vi "UUT Test Info Update Cycle Count.vi"(11 "Sequence Context":T1) -> (0 "error out":errorcluster)   [LabVIEW 2023, in "HardwareAbstractionLayer_LVOOP.lvlib" / "Report.lvclass"]
uses:
  Report.lvclass
  <vilib>/addons/TestStand/_TSLegacy.llb/LabVIEW Test - Sequence Context.ctl
  Database/SQL Public VI/Control/DB Options.ctl
  <vilib>/addons/TestStand/_TSUtility.llb/TestStand - Get Property Value (Number {Unsigned 32-bit Integer}).vi
  Database/Database.lvclass
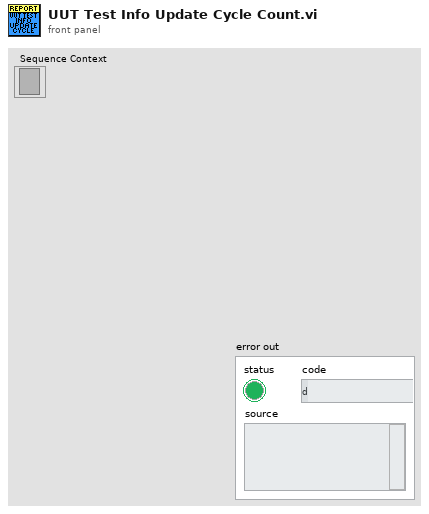
[diagram p1: front panel]
types:
  T1 = typedef "LabVIEW Test - Sequence Context.ctl" = refnum<k7>
  T2 = typedef "HardwareAbstractionLayer_LVOOP.lvlib/Database.lvclass/DB Options.ctl" = enum16{"Init", "Select Data", "Insert Data", "Update Data", "Delete Data", "Execute Query", "Create Schema", "Create Table", "List Tables", "List Columns", "Close"}
  T3 = typedef "HardwareAbstractionLayer_LVOOP.lvlib/Report.lvclass/Result FGV Data.ctl" = cluster{"Project Name":string, "Product Name":string, "Product Varient":string, "Test Name":string, "Test Phase":string, "Test Description":string, "Temp Chamber Name":string, "Schema":string, "Total No of Cycles":u32, "Current Cycle Number":u32, "Cycle Duration":u32, "Current Test Mode":string}
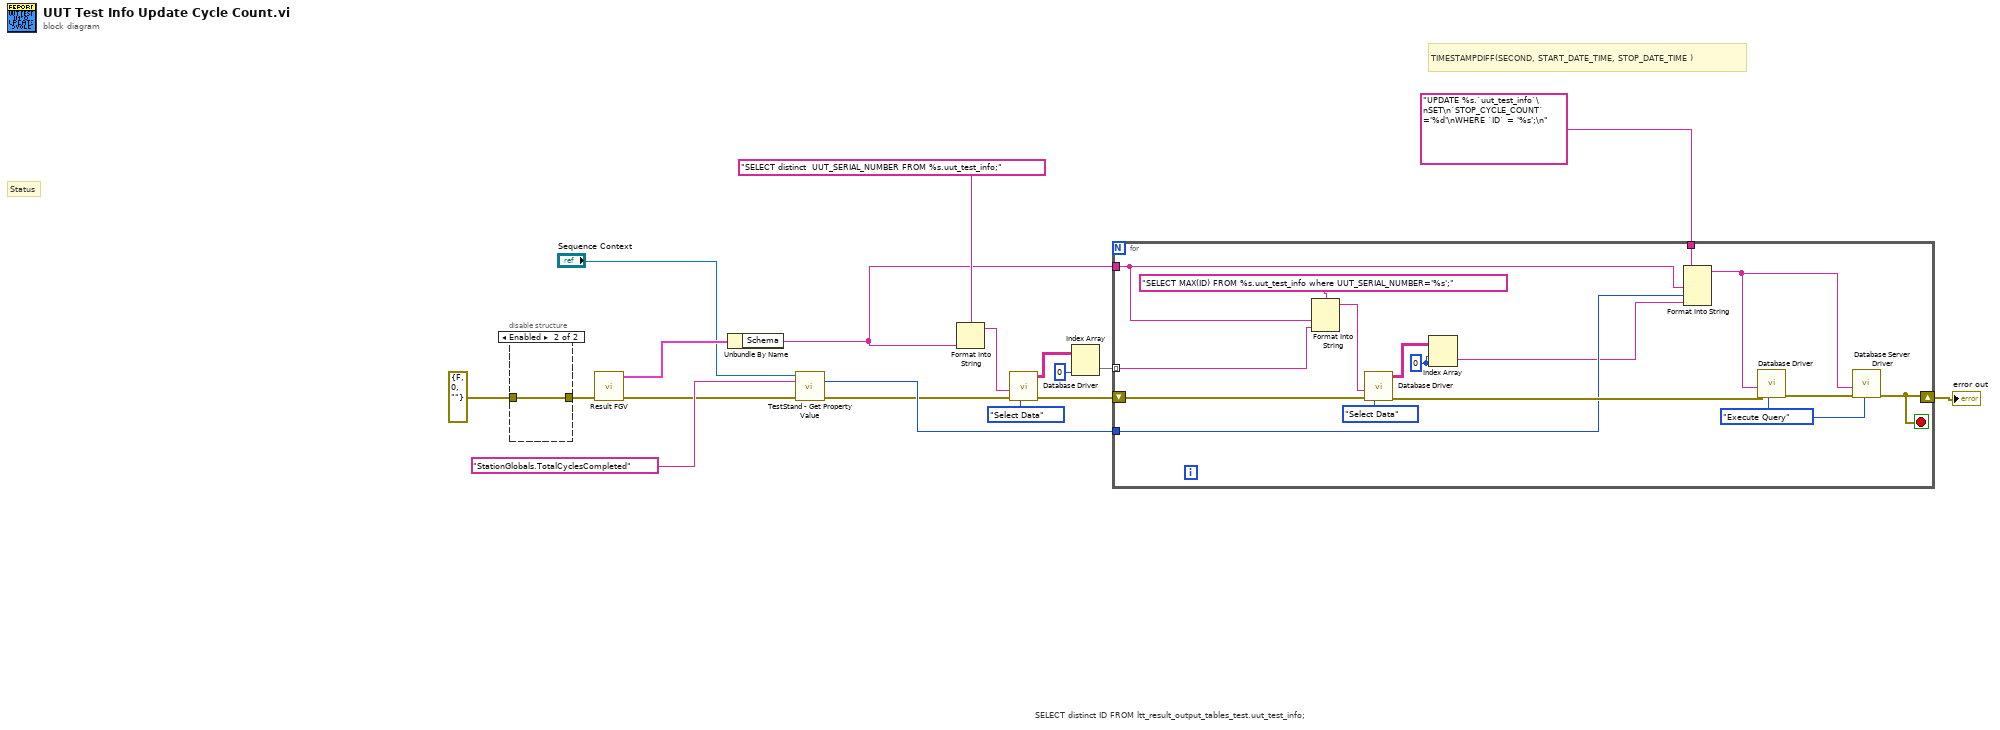
[diagram p0: block diagram]
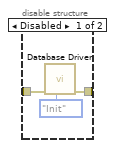
[diagram p2: hidden frame]
diagram:
  # "TIMESTAMPDIFF(SECOND, START_DATE_TIME, STOP_DATE_TIME )"
  # "Status"
  # "SELECT distinct ID FROM ltt_result_output_tables_test.uut_test_info;"
  n1 = disable-structure shown="Enabled" {
    disable-tunnel: errorcluster {"status"=FALSE, "code"=0, "source"=""} ("error in") -> [w20 w22]
    disable-tunnel: [w19 w22] -> w15
    frame Disabled {
      n2 = call "Database Driver.vi"("Options"=DB_Options."Init", "error in"=w20) -> ("error out"=w19:errorcluster)  [unwired: 6 in, 3 out]
    }
    frame Enabled {
    }
  }
  n3 = call "Result FGV.vi"("error in"=w15) -> ("error out"=w3:errorcluster, "Result FGV Data Out"=w17:T3)  [unwired: 9 in]
  n4 = Unbundle By Name(w17) -> ("Schema"=w9:string)
  n5 = call-poly <vilib>:"TestStand - Get Property Value.vi"("Sequence Context In"="Sequence Context", "Lookup String"="StationGlobals.TotalCyclesCompleted", "error in (no error)"=w3) -> ("Value"=w2:u32, "error out"=w1:errorcluster)  [unwired: 10 in, 1 out]
  n6 = Format Into String(format string="SELECT distinct  UUT_SERIAL_NUMBER FROM %s.uut_test_info;", w9) -> (resulting string=w10:string)  [unwired: 2 in, 1 out]
  n7 = call "Database Driver.vi"("Options"=DB_Options."Select Data", "error in"=w1, "SQL query"=w10) -> ("error out"=w12:errorcluster, "data"=w8:string[][])  [unwired: 5 in, 2 out]
  n8 = Index Array(array=w8, index (col)=0 ("disabled index (col)")) -> (element=w6:string[])  [unwired: 1 in]
  n9 = for {
    tunnel: w9 -> [w31]
    shift-right: [w25] -> w18
    shift-left: w12 -> [w36]
    tunnel: "UPDATE %s.`uut_test_info`\nSET\n`STOP_CYCLE_COUNT` ='%d'\nWHERE `ID` = '%s';\n" ("format string") -> [w32]
    tunnel: w2 -> [w29]
    tunnel: w6 -> [w27] mode=indexing
    stop <- w25 stop-if-true
    w23 = DB_Options."Execute Query" ("Options")
    w30 = 0 ("disabled index (col)")
    n10 = Format Into String(format string="SELECT MAX(ID) FROM %s.uut_test_info where UUT_SERIAL_NUMBER='%s';", w31, w27) -> (resulting string=w37:string)  [unwired: 2 in, 1 out]
    n11 = call "Database Driver.vi"("Options"=DB_Options."Select Data", "error in"=w36, "SQL query"=w37) -> ("error out"=w33:errorcluster, "data"=w35:string[][])  [unwired: 5 in, 2 out]
    n12 = Index Array(array=w35, index (row)=w30, index (col)=w30) -> (element=w28:string)
    n13 = Format Into String(format string=w32, w31, w29, w28) -> (resulting string=w24:string)  [unwired: 2 in, 1 out]
    n14 = call "Database Driver.vi"("Options"=w23, "error in"=w33, "SQL query"=w24) -> ("error out"=w26:errorcluster)  [unwired: 5 in, 3 out]
    n15 = call "Database Server Driver.vi"("Options"=w23, "error in"=w26, "SQL query"=w24) -> ("error out"=w25:errorcluster)  [unwired: 5 in, 3 out]
  }
  "error out" <- w18
